vi "hostVI.vi"() -> ()   [LabVIEW 2017]
uses:
  <vilib>/rvi/interface/nirviOpenFPGA/nirviOpenFPGA.xnode
  targetVI.vi
  <vilib>/rvi/interface/nirviReadWriteControl/nirviReadWriteControl.xnode
  <vilib>/rvi/interface/nirviCloseFPGA/nirviCloseFPGA.xnode
  <vilib>/rvi/interface/nirviMethod/nirviMethod.xnode
  <vilib>/FPGAPlugInAG/Dynamic/niLvFpga_Run_Dynamic.vi
  <vilib>/rvi/interface/Simulation/niFpgaSimulationCallBeginRW.vi
  <vilib>/rvi/errors/niLvFpgaAdjustHostInterfaceError.vi
  <vilib>/FPGAPlugInAG/Dynamic/niLvFpga_AcquireReadRegionFifo_Dynamic.vi
  <vilib>/rvi/errors/niLvFpgaMergeErrorWithErrorCode.vi
  <vilib>/FPGAPlugInAG/Dynamic/niLvFpga_Close_Dynamic.vi
  <vilib>/rvi/interface/RandomDataEmulation/nirviRandomDataOpen.vi
  <vilib>/rvi/interface/common/niFpgaCacheSessionInfoDynamic.vi
panel:
  out "Elements Remaining":u32
  out "Elements In Region":u32
  out "Read Region Reference":refnum<data-value>
  in  "Timeout (ms)":i32=5000
  in  "Number of Elements":u32
  in  "end point":fxp<+/-,16,16>
  in  "start point":fxp<+/-,16,16>
  in  "update time":fxp<+,16,16>
  in  "N pts in waveform":fxp<+/-,16,16>
  in  "Boolean":bool
  out "y":fxp<+/-,16,16>
  in  "stop":bool
  out "error out":errorcluster
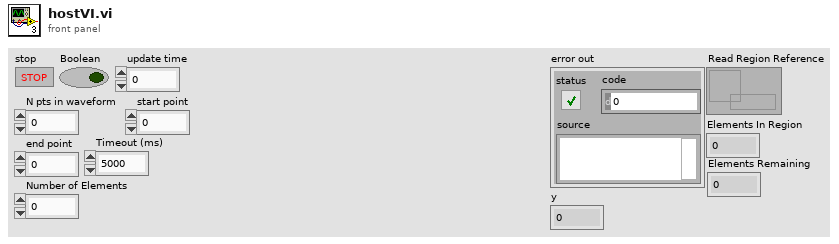
[diagram p1: front panel]
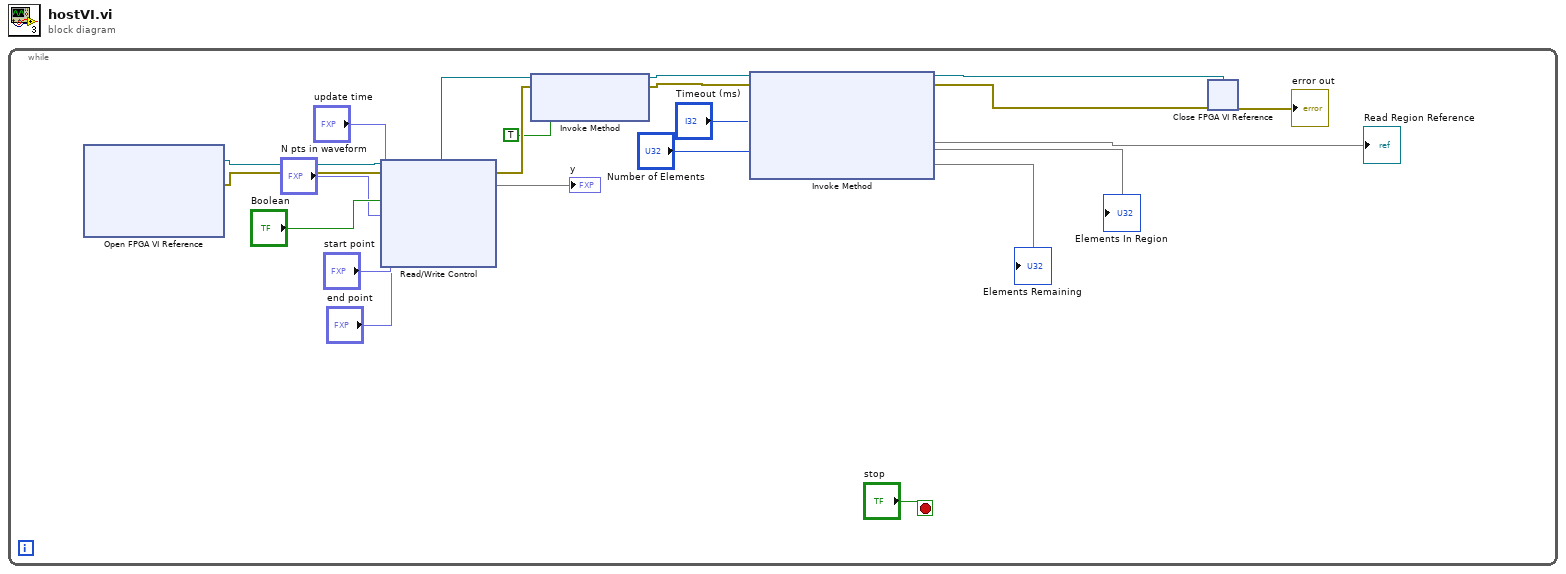
[diagram p0: block diagram]
diagram:
  n1 = while {
    stop <- "stop" stop-if-true
    n2 = xnode "Open FPGA VI Reference"() -> ("FPGA VI Reference Out"=w22:refnum<k20>, "error out"=w21:errorcluster)  [unwired: 2 in]
    n3 = xnode "Read/Write Control"("FPGA VI Reference In"=w22, "error in"=w21, "Boolean"="Boolean", "N pts in waveform"="N pts in waveform", "update time"="update time", "start point"="start point", "end point"="end point") -> ("FPGA VI Reference Out"=w19:refnum<k20>, "error out"=w18:errorcluster, "y"=→"y")
    n4 = xnode "Invoke Method"("FPGA VI Reference In"=w19, "error in"=w18, "Wait Until Done (F)"=TRUE) -> ("FPGA VI Reference Out"=w10:refnum<k20>, "error out"=w9:errorcluster)
    n5 = xnode "Invoke Method"("FPGA VI Reference In"=w10, "error in"=w9, "Number of Elements"="Number of Elements", "Timeout (ms)"="Timeout (ms)") -> ("FPGA VI Reference Out"=w8:refnum<k20>, "error out"=w7:errorcluster, "Read Region Reference"=→"Read Region Reference", "Elements in Region"=→"Elements In Region", "Elements Remaining"=→"Elements Remaining")
    n6 = xnode "Close FPGA VI Reference"("FPGA VI Reference In"=w8, "error in"=w7) -> ("error out"=→"error out":errorcluster)
  }
